vi "CI_IMAQ_AdjustBeadPos.vi"(9 "Corner-based bead pos":cluster{"X":i32, "Y":i32}[](array[cluster]), 11 "Camera state":variant) -> (1 "Adjusted bead pos (out)":cluster{"X":i32, "Y":i32}[](array[cluster]), 3 "Camera state (out)":variant)   [LabVIEW 2011]
uses:
  GenericIMAQCameraInstance.ctl
  Main/Camera/GenericCameraConfigType.ctl
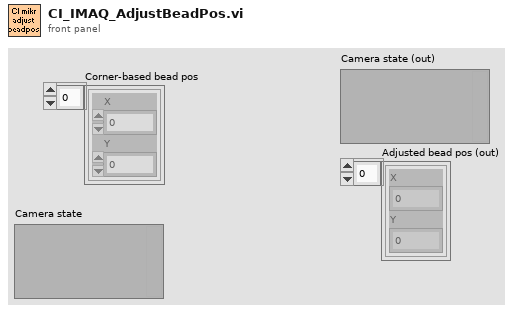
[diagram p1: front panel]
types:
  T1 = typedef "GenericIMAQCameraInstance.ctl" = cluster{"Session":refnum<k11>, "Settings":T2}
  T2 = typedef "GenericCameraConfigType.ctl" = cluster{"Framerate (Hz)":i32, "Exposure time (us)":i32, "Image size":cluster{"Width":i32, "Height":i32}, "Number of buffers":i32}
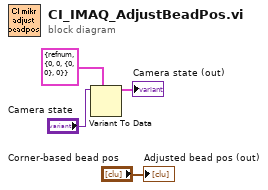
[diagram p0: block diagram]
diagram:
  n1 = Variant To Data(type=T1 {"Session"=refnum, "Settings"={"Framerate (Hz)"=0, "Exposure time (us)"=0, "Image size"={"Width"=0, "Height"=0}, "Number of buffers"=0}} ("Generic IMAQ Camera Instance"), Variant="Camera state") -> (data=→"Camera state (out)":T1)  [unwired: 1 in, 1 out]
  "Adjusted bead pos (out)" <- "Corner-based bead pos"
